vi "Straight_MotorControl_r1 (SubVI).vi"(6 "Goal Y Coord":dbl, 9 "Goal X Coord":dbl, 10 "Current Y Pos":dbl, 11 "Current X Pos":dbl) -> (2 "Output Velocity Gain":dbl, 3 "Numeric Out Y":dbl)   [LabVIEW 2015]
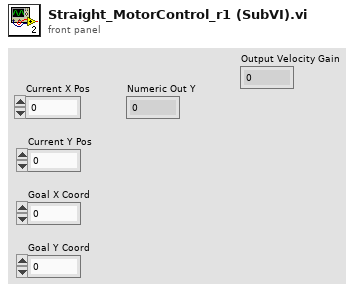
[diagram p1: front panel]
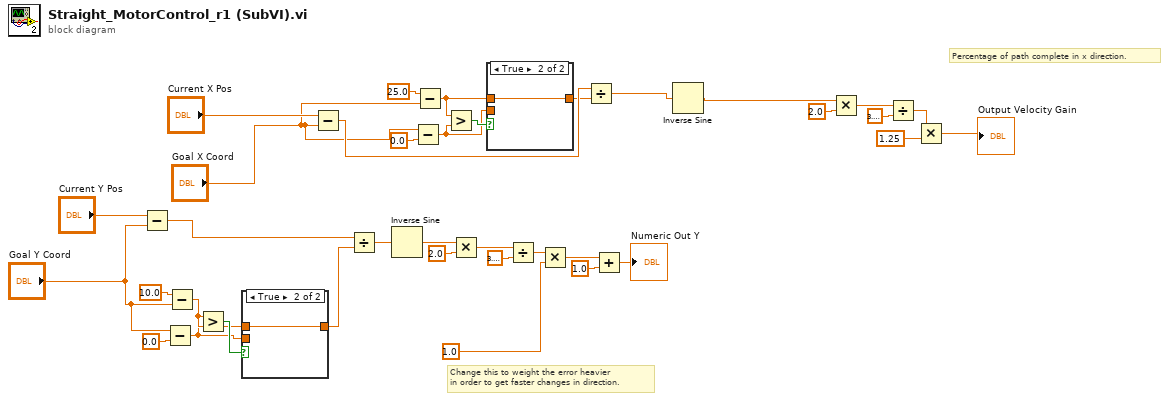
[diagram p0: block diagram]
diagram:
  # "Percentage of path complete in x direction."
  # "Change this to weight the error heavier\nin order to get faster changes in direction."
  n1 = Subtract(x="Current Y Pos", y="Goal Y Coord") -> (x-y=w26:dbl)
  n2 = Subtract(x="Goal Y Coord", y=0.0 ("x")) -> (x-y=w2:dbl)
  n3 = Subtract(x=10.0, y="Goal Y Coord") -> (x-y=w3:dbl)
  n4 = Greater?(x=w3, y=w2) -> (0:w4:bool)
  n5 = case shown="True" w4 {
    tunnel: w3 -> [_ w38]
    tunnel: [w37 w38] -> w1
    tunnel: w2 -> [w37 _]
    frame False {
    }
    frame True {
    }
  }
  n6 = Subtract(x="Current X Pos", y="Goal X Coord") -> (x-y=w25:dbl)
  n7 = Divide(x=w26, y=w1) -> (x/y=w27:dbl)
  n8 = Inverse Sine(1:w27) -> (0:w28:dbl)
  n9 = Subtract(x="Goal X Coord", y=0.0 ("x")) -> (x-y=w17:dbl)
  n10 = Subtract(x=25.0, y="Goal X Coord") -> (x-y=w18:dbl)
  n11 = Greater?(x=w18, y=w17) -> (0:w19:bool)
  n12 = Multiply(x=w28, y=2.0) -> (x*y=w30:dbl)
  n13 = case shown="True" w19 {
    tunnel: w18 -> [_ w40]
    tunnel: [w39 w40] -> w15
    tunnel: w17 -> [w39 _]
    frame False {
    }
    frame True {
    }
  }
  n14 = Divide(x=w30, y=3.141592653589793) -> (x/y=w33:dbl)
  n15 = Multiply(x=w33, y=1.0) -> (x*y=w34:dbl)
  n16 = Divide(x=w25, y=w15) -> (x/y=w14:dbl)
  n17 = Add(x=w34, y=1.0) -> (x+y=→"Numeric Out Y":dbl)
  n18 = Inverse Sine(1:w14) -> (0:w10:dbl)
  n19 = Multiply(x=w10, y=2.0) -> (x*y=w12:dbl)
  n20 = Divide(x=w12, y=3.141592653589793) -> (x/y=w9:dbl)
  n21 = Multiply(x=w9, y=1.25) -> (x*y=→"Output Velocity Gain":dbl)
